vi "set RF board amplitude - interlace.vi"(1 "Board 2 Amplitude Limits":T1={"Minimum"=0.0, "Maximum"=50.0, "Increment"=1.0}, 2 "Board 1 Amplitude Limits":T1={"Minimum"=0.0, "Maximum"=50.0, "Increment"=1.0}, 4 "error in":errorcluster, 5 "FPGA VI Reference In":T2, 6 "Board 2 Amplitude 3 (%)":dbl, 7 "Board 1 Amplitude 3 (%)":dbl, 8 "Board 2 Amplitude 2 (%)":dbl, 9 "Board 2 Amplitude 1 (%)":dbl, 10 "Board 1 Amplitude 2 (%)":dbl, 11 "Board 1 Amplitude 1 (%)":dbl) -> (0 "error out":errorcluster, 3 "FPGA VI Reference Out":T2)   [LabVIEW 2014]
uses:
  <vilib>/rvi/interface/nirviReadWriteControl/nirviReadWriteControl.xnode
  openfpgaref.8.6.ctl
  C:/Users/temp/Desktop/labview UHR-Fleezers instrument control/FPGA Bitfiles/UHR-FleezersInst_FPGATarget_UHR-FleezersCont_I9m189Wk6wg.lvbitx
  C:/Users/temp/Desktop/labview UHR-Fleezers instrument control/UHR-Fleezers Control (fpga) - 10.9.vi
  NiFpgaLv.dll
  <vilib>/Utility/error.llb/Error Cluster From Error Code.vi
  <vilib>/rvi/errors/niLvFpgaAdjustHostInterfaceError.vi
  <vilib>/Utility/miscctls.llb/LVMinMaxIncTypeDef.ctl
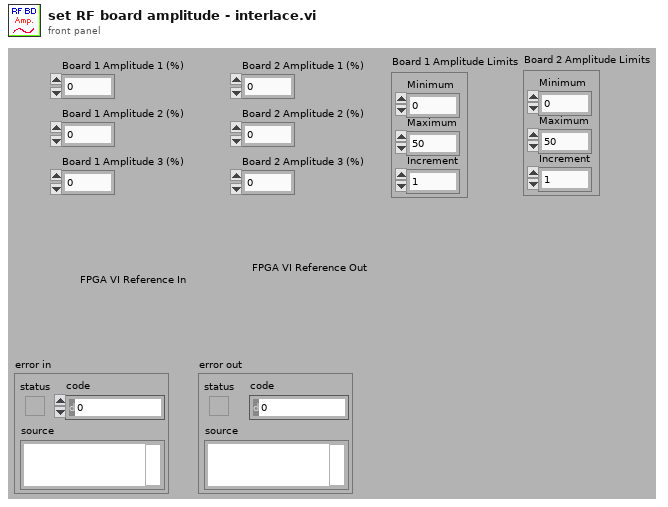
[diagram p1: front panel]
types:
  T1 = typedef "LVMinMaxIncTypeDef.ctl" = cluster{"Minimum":dbl, "Maximum":dbl, "Increment":dbl}
  T2 = typedef "openfpgaref.8.6.ctl" = refnum<k20>
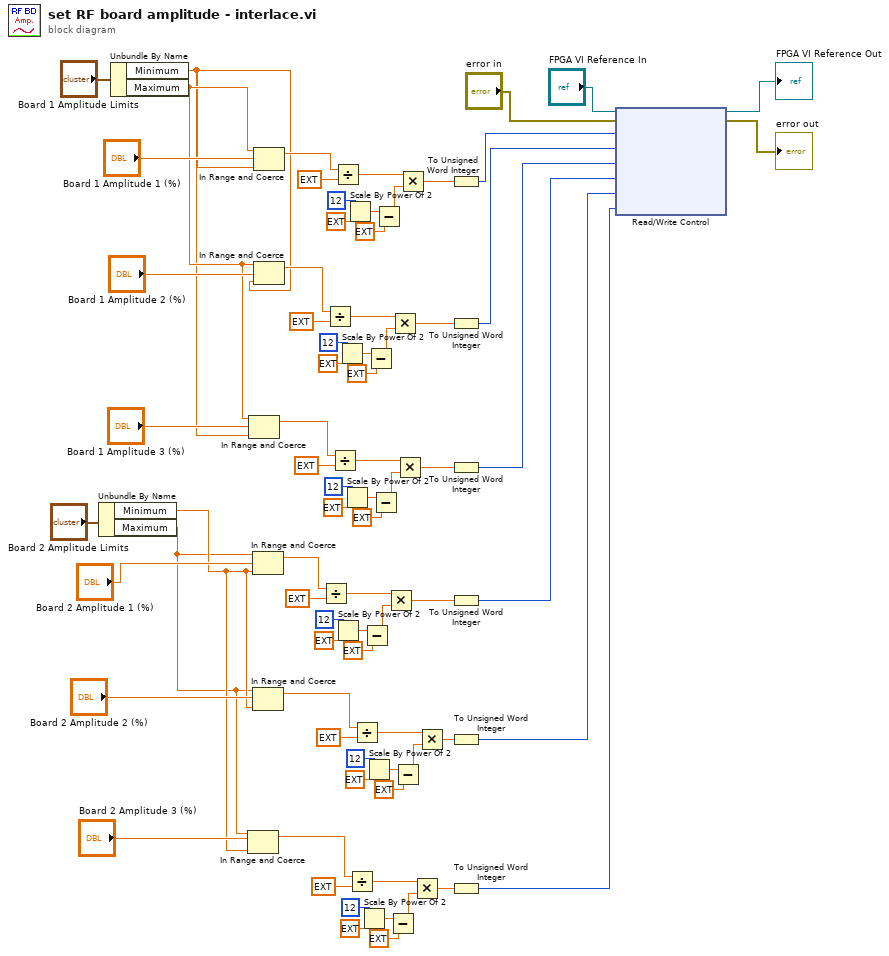
[diagram p0: block diagram]
diagram:
  n1 = Unbundle By Name("Board 2 Amplitude Limits") -> ("Minimum"=w2:dbl, "Maximum"=w1:dbl)
  n2 = Unbundle By Name("Board 1 Amplitude Limits") -> ("Minimum"=w3:dbl, "Maximum"=w4:dbl)
  n3 = In Range and Coerce(upper limit=w1, x="Board 2 Amplitude 3 (%)", lower limit=w2) -> (coerced(x)=w14:dbl)  [unwired: 1 out]
  n4 = In Range and Coerce(upper limit=w4, x="Board 1 Amplitude 3 (%)", lower limit=w3) -> (coerced(x)=w16:dbl)  [unwired: 1 out]
  n5 = In Range and Coerce(upper limit=w1, x="Board 2 Amplitude 1 (%)", lower limit=w2) -> (coerced(x)=w17:dbl)  [unwired: 1 out]
  n6 = In Range and Coerce(upper limit=w1, x="Board 2 Amplitude 2 (%)", lower limit=w2) -> (coerced(x)=w18:dbl)  [unwired: 1 out]
  n7 = In Range and Coerce(upper limit=w4, x="Board 1 Amplitude 1 (%)", lower limit=w3) -> (coerced(x)=w21:dbl)  [unwired: 1 out]
  n8 = In Range and Coerce(upper limit=w4, x="Board 1 Amplitude 2 (%)", lower limit=w3) -> (coerced(x)=w19:dbl)  [unwired: 1 out]
  n9 = Divide(x=w17, y=ext 100.0) -> (x/y=w44:ext)
  n10 = Divide(x=w19, y=ext 100.0) -> (x/y=w60:ext)
  n11 = Divide(x=w16, y=ext 100.0) -> (x/y=w52:ext)
  n12 = Divide(x=w21, y=ext 100.0) -> (x/y=w68:ext)
  n13 = Scale By Power Of 2(n=i16 12, x=ext 1.0) -> (x*2^n=w47:ext)
  n14 = Scale By Power Of 2(n=i16 12, x=ext 1.0) -> (x*2^n=w63:ext)
  n15 = Scale By Power Of 2(n=i16 12, x=ext 1.0) -> (x*2^n=w55:ext)
  n16 = Scale By Power Of 2(n=i16 12, x=ext 1.0) -> (x*2^n=w71:ext)
  n17 = Divide(x=w14, y=ext 100.0) -> (x/y=w28:ext)
  n18 = Divide(x=w18, y=ext 100.0) -> (x/y=w36:ext)
  n19 = Scale By Power Of 2(n=i16 12, x=ext 1.0) -> (x*2^n=w31:ext)
  n20 = Subtract(x=w47, y=ext 1.0) -> (x-y=w45:ext)
  n21 = Scale By Power Of 2(n=i16 12, x=ext 1.0) -> (x*2^n=w39:ext)
  n22 = Subtract(x=w63, y=ext 1.0) -> (x-y=w61:ext)
  n23 = Subtract(x=w55, y=ext 1.0) -> (x-y=w53:ext)
  n24 = Subtract(x=w71, y=ext 1.0) -> (x-y=w69:ext)
  n25 = Multiply(x=w44, y=w45) -> (x*y=w43:ext)
  n26 = Subtract(x=w31, y=ext 1.0) -> (x-y=w29:ext)
  n27 = Multiply(x=w60, y=w61) -> (x*y=w59:ext)
  n28 = Subtract(x=w39, y=ext 1.0) -> (x-y=w37:ext)
  n29 = Multiply(x=w52, y=w53) -> (x*y=w51:ext)
  n30 = Multiply(x=w68, y=w69) -> (x*y=w67:ext)
  n31 = Multiply(x=w28, y=w29) -> (x*y=w27:ext)
  n32 = Multiply(x=w36, y=w37) -> (x*y=w35:ext)
  n33 = To Unsigned Word Integer(number=w67) -> (unsigned 16bit integer=w10:u16)
  n34 = To Unsigned Word Integer(number=w59) -> (unsigned 16bit integer=w9:u16)
  n35 = To Unsigned Word Integer(number=w51) -> (unsigned 16bit integer=w8:u16)
  n36 = To Unsigned Word Integer(number=w43) -> (unsigned 16bit integer=w7:u16)
  n37 = To Unsigned Word Integer(number=w35) -> (unsigned 16bit integer=w6:u16)
  n38 = To Unsigned Word Integer(number=w27) -> (unsigned 16bit integer=w5:u16)
  n39 = xnode ("Read/Write Control")("FPGA VI Reference In"="FPGA VI Reference In", "error in"="error in", "BD 1 Amplitude 1"=w10, "BD 1 Amplitude 2"=w9, "BD 1 Amplitude 3"=w8, "BD 2 Amplitude 1"=w7, "BD 2 Amplitude 2"=w6, "BD 2 Amplitude 3"=w5) -> ("FPGA VI Reference Out"=→"FPGA VI Reference Out":T2, "error out"=→"error out":errorcluster)
